vi "LDA_U16_data_header.vi"() -> (0 "Output string":string)   [LabVIEW 2010]
uses:
  Globals/Meas_global.vi
  Globals/LDA_meas_global_1.vi
  Globals/LDA_meas_global_2.vi
panel:
  out "length":i32
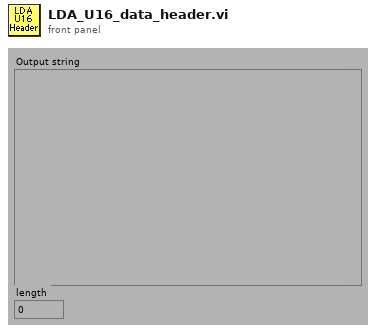
[diagram p1: front panel]
types:
  T1 = typedef "BSA_info_Cluster.ctl" = cluster{"GPIB Address":string, "No of Check Bytes":i32, "Extra Info":string, "COLOUR":u32, "Wavelength (nm)":dbl}
  T2 = typedef "BSA_Type.ctl" = enum16{"57N11", "BSA F60"}
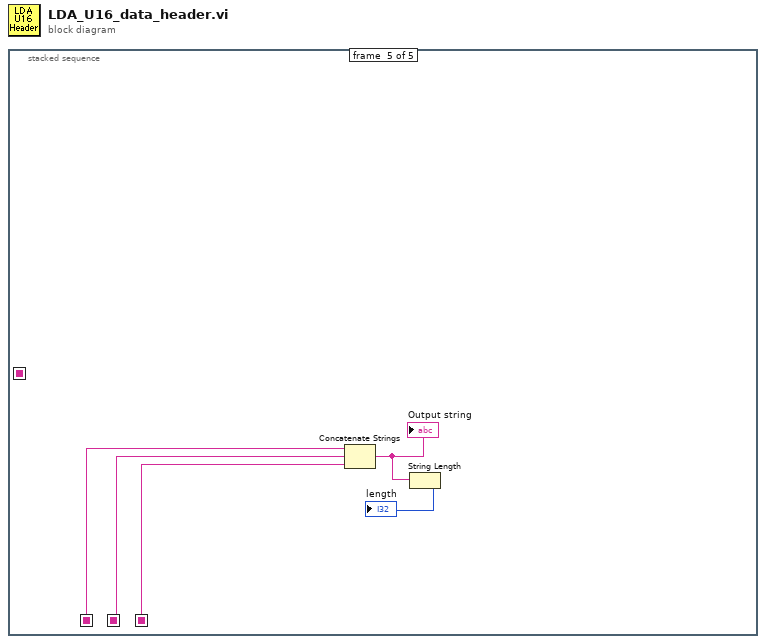
[diagram p0: block diagram]
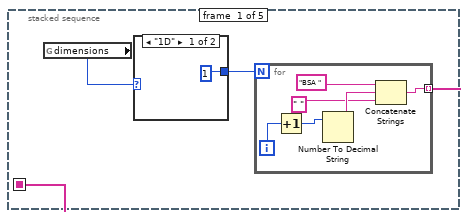
[diagram p2: hidden frame]
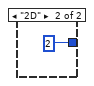
[diagram p3: hidden frame]
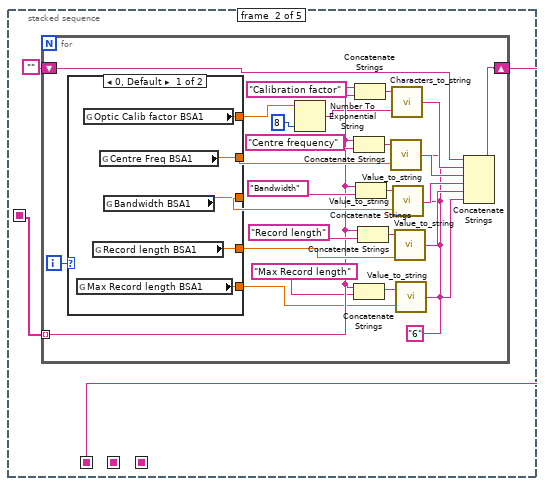
[diagram p4: hidden frame]
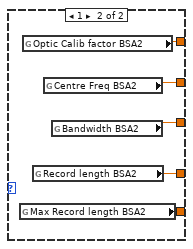
[diagram p5: hidden frame]
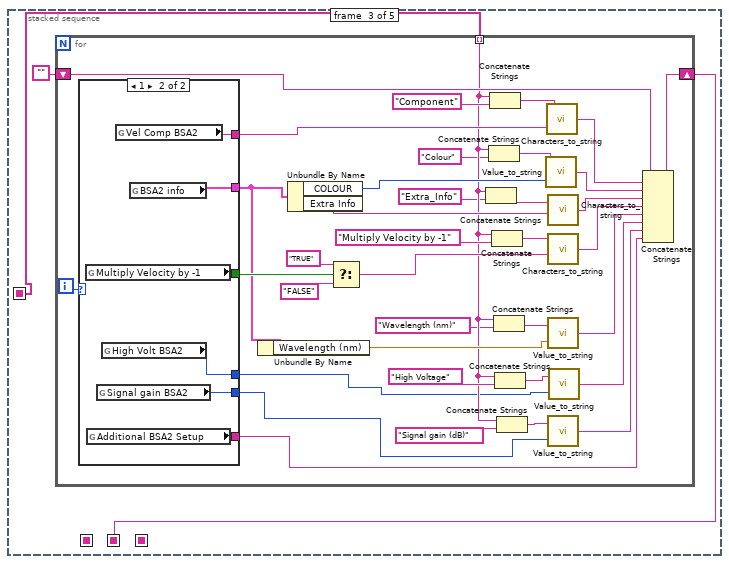
[diagram p6: hidden frame]
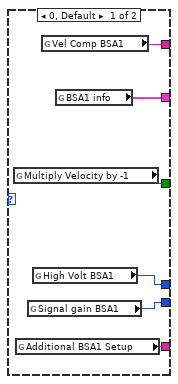
[diagram p7: hidden frame]
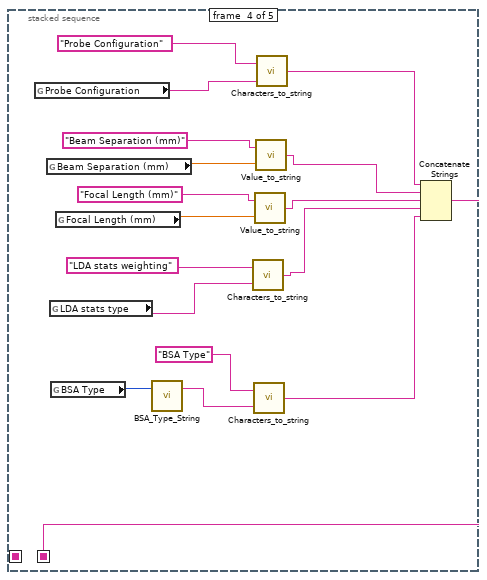
[diagram p8: hidden frame]
diagram:
  n1 = stacked-sequence {
    seq-local: [_ w13 _ _ _] -> [_ _ _ _ w125]
    seq-local: [_ _ w53 _ _] -> [_ _ _ _ w124]
    seq-local: [w3 _ _ _ _] -> [_ w12 w52 _ _]
    seq-local: [_ _ _ w117 _] -> [_ _ _ _ w121]
    frame #0 {
      n2 = global read "Meas_global.vi" "dimensions"() -> (w2:enum16{"1D", "2D"})
      n3 = case shown="\"1D\"" w2 {
        tunnel: [1 2] -> w1
        frame "1D" {
        }
        frame "2D" {
        }
      }
      n4 = for {
        N: w1 -> [_]
        tunnel: [w8] -> w3 mode=indexing
        i -> [w6]
        n5 = Increment(x=w6) -> (x+1=w9:i32)
        n6 = Number To Decimal String(number=w9) -> (decimal integer string=w11:string)  [unwired: 1 out]
        n7 = Concatenate Strings("BSA ", w11, " ") -> (w8:string)
      }
    }
    frame #1 {
      n8 = for {
        shift-right: [w39] -> w13
        shift-left: "" -> [w40]
        tunnel: w12 -> [w23] mode=indexing
        i -> [w41]
        w18 = "6" ("precision")
        n9 = case shown="0, Default" w41 {
          tunnel: [w46 w48] -> w16
          tunnel: [w45 w49] -> w32
          tunnel: [w44 w50] -> w33
          tunnel: [w43 w51] -> w34
          tunnel: [w42 w47] -> w20
          frame 0, Default {
            n10 = global read "LDA_meas_global_1.vi" "Max Record length BSA1"() -> (w42:dbl)
            n11 = global read "LDA_meas_global_1.vi" "Optic Calib factor BSA1"() -> (w46:dbl)
            n12 = global read "LDA_meas_global_1.vi" "Record length BSA1"() -> (w43:dbl)
            n13 = global read "LDA_meas_global_1.vi" "Centre Freq BSA1"() -> (w45:dbl)
            n14 = global read "LDA_meas_global_1.vi" "Bandwidth BSA1"() -> (w44:dbl)
          }
          frame 1 {
            n15 = global read "LDA_meas_global_2.vi" "Max Record length BSA2"() -> (w47:dbl)
            n16 = global read "LDA_meas_global_2.vi" "Optic Calib factor BSA2"() -> (w48:dbl)
            n17 = global read "LDA_meas_global_2.vi" "Record length BSA2"() -> (w51:dbl)
            n18 = global read "LDA_meas_global_2.vi" "Centre Freq BSA2"() -> (w49:dbl)
            n19 = global read "LDA_meas_global_2.vi" "Bandwidth BSA2"() -> (w50:dbl)
          }
        }
        n20 = Number To Exponential String(number=w16, precision (6)=i16 8) -> (E-format string=w15:string)  [unwired: 2 out]
        n21 = Concatenate Strings(w23, "Centre frequency") -> (w37:string)
        n22 = Concatenate Strings(w23, "Max Record length") -> (w21:string)
        n23 = Concatenate Strings(w23, "Calibration factor") -> (w38:string)
        n24 = Concatenate Strings(w23, "Bandwidth") -> (w36:string)
        n25 = Concatenate Strings(w23, "Record length") -> (w35:string)
        n26 = call "Value_to_string.vi"("precision"=w18, "Value"=w32, "Label for value"=w37) -> ("Output string"=w30:string)
        n27 = call "Characters_to_string.vi"("Characters to write"=w15, "Label for characters"=w38) -> ("Output string"=w31:string)
        n28 = call "Value_to_string.vi"("precision"=w18, "Value"=w33, "Label for value"=w36) -> ("Output string"=w29:string)
        n29 = call "Value_to_string.vi"("precision"=w18, "Value"=w34, "Label for value"=w35) -> ("Output string"=w24:string)
        n30 = call "Value_to_string.vi"("precision"=w18, "Value"=w20, "Label for value"=w21) -> ("Output string"=w19:string)
        n31 = Concatenate Strings(w40, w31, w30, w29, w24, w19) -> (w39:string)
      }
    }
    frame #2 {
      n32 = for {
        shift-right: [w89] -> w53
        shift-left: "" -> [w90]
        tunnel: w52 -> [w64] mode=indexing
        i -> [w91]
        n33 = case shown="1" w91 {
          tunnel: [w97 w103] -> w71
          tunnel: [w96 w102] -> w82
          tunnel: [w95 w101] -> w79
          tunnel: [w93 w100] -> w57
          tunnel: [w94 w99] -> w56
          tunnel: [w92 w98] -> w55
          frame 0, Default {
            n34 = global read "LDA_meas_global_1.vi" "Multiply Velocity by -1"() -> (w95:bool)
            n35 = global read "LDA_meas_global_1.vi" "Additional BSA1 Setup"() -> (w92:string)
            n36 = global read "LDA_meas_global_1.vi" "Signal gain BSA1"() -> (w93:i16)
            n37 = global read "LDA_meas_global_1.vi" "High Volt BSA1"() -> (w94:i16)
            n38 = global read "LDA_meas_global_1.vi" "Vel Comp BSA1"() -> (w96:string)
            n39 = global read "LDA_meas_global_1.vi" "BSA1 info"() -> (w97:T1)
          }
          frame 1 {
            n40 = global read "LDA_meas_global_2.vi" "Multiply Velocity by -1"() -> (w101:bool)
            n41 = global read "LDA_meas_global_2.vi" "Additional BSA2 Setup"() -> (w98:string)
            n42 = global read "LDA_meas_global_2.vi" "Signal gain BSA2"() -> (w100:i16)
            n43 = global read "LDA_meas_global_2.vi" "High Volt BSA2"() -> (w99:i16)
            n44 = global read "LDA_meas_global_2.vi" "Vel Comp BSA2"() -> (w102:string)
            n45 = global read "LDA_meas_global_2.vi" "BSA2 info"() -> (w103:T1)
          }
        }
        n46 = Unbundle By Name(w71) -> ("Wavelength (nm)"=w70:dbl)
        n47 = Unbundle By Name(w71) -> ("COLOUR"=w84:u32, "Extra Info"=w73:string)
        n48 = Select(t="TRUE" ("y"), s=w79, f="FALSE" ("y")) -> (s? t:f=w76:string)
        n49 = Concatenate Strings(w64, "Extra_Info" ("string")) -> (w72:string)
        n50 = Concatenate Strings(w64, "Colour") -> (w87:string)
        n51 = Concatenate Strings(w64, "Component") -> (w88:string)
        n52 = Concatenate Strings(w64, "Multiply Velocity by -1") -> (w80:string)
        n53 = Concatenate Strings(w64, "Wavelength (nm)") -> (w69:string)
        n54 = Concatenate Strings(w64, "High Voltage") -> (w68:string)
        n55 = Concatenate Strings(w64, "Signal gain (dB)") -> (w67:string)
        n56 = call "Value_to_string.vi"("Value"=w84, "Label for value"=w87) -> ("Output string"=w85:string)  [unwired: 1 in]
        n57 = call "Characters_to_string.vi"("Characters to write"=w82, "Label for characters"=w88) -> ("Output string"=w86:string)
        n58 = call "Characters_to_string.vi"("Characters to write"=w73, "Label for characters"=w72) -> ("Output string"=w74:string)
        n59 = call "Characters_to_string.vi"("Characters to write"=w76, "Label for characters"=w80) -> ("Output string"=w75:string)
        n60 = call "Value_to_string.vi"("Value"=w70, "Label for value"=w69) -> ("Output string"=w61:string)  [unwired: 1 in]
        n61 = call "Value_to_string.vi"("Value"=w57, "Label for value"=w67) -> ("Output string"=w63:string)  [unwired: 1 in]
        n62 = call "Value_to_string.vi"("Value"=w56, "Label for value"=w68) -> ("Output string"=w62:string)  [unwired: 1 in]
        n63 = Concatenate Strings(w90, w86, w85, w74, w75, w61, w62, w63, w55) -> (w89:string)
      }
    }
    frame #3 {
      n64 = global read "LDA_meas_global_1.vi" "Probe Configuration"() -> (w116:string)
      n65 = global read "LDA_meas_global_1.vi" "Beam Separation (mm)"() -> (w115:dbl)
      n66 = global read "LDA_meas_global_1.vi" "LDA stats type"() -> (w119:string)
      n67 = global read "LDA_meas_global_1.vi" "BSA Type"() -> (w107:T2)
      n68 = global read "LDA_meas_global_1.vi" "Focal Length (mm)"() -> (w114:dbl)
      n69 = call "BSA_Type_String.vi"("BSA Type"=w107) -> ("BSA String Out"=w106:string)  [unwired: 1 in, 1 out]
      n70 = call "Characters_to_string.vi"("Characters to write"=w119, "Label for characters"="LDA stats weighting") -> ("Output string"=w108:string)
      n71 = call "Characters_to_string.vi"("Characters to write"=w106, "Label for characters"="BSA Type") -> ("Output string"=w105:string)
      n72 = call "Value_to_string.vi"("Value"=w114, "Label for value"="Focal Length (mm)" ("Label for characters")) -> ("Output string"=w109:string)  [unwired: 1 in]
      n73 = call "Value_to_string.vi"("Value"=w115, "Label for value"="Beam Separation (mm)" ("Label for characters")) -> ("Output string"=w110:string)  [unwired: 1 in]
      n74 = call "Characters_to_string.vi"("Characters to write"=w116, "Label for characters"="Probe Configuration") -> ("Output string"=w111:string)
      n75 = Concatenate Strings(w111, w110, w109, w108, w105) -> (w117:string)
    }
    frame #4 {
      n76 = Concatenate Strings(w125, w124, w121) -> (w122:string)
      "Output string" <- w122
      n77 = String Length(string=w122) -> (length=→"length":i32)
    }
  }
